vi "Simple Serial.vi"() -> ()   [LabVIEW 2018]
doc: "This example performs a serial port write and a serial port read. The parameters set for the serial port must match the parameters of the connected instrument or device. The VISA Configure Serial Port VI sets the configuration parameters. The front panel displays the controls used to configure the basic parameters, such as baud rate, data bits, and parity. The VI passes the VISA resource name to other VIs that perform operations on that VISA resource. The VISA Write function sends a command to the serial device and the VISA Read function returns data based on the command. The VISA Close function then closes the reference to the serial device. It is important to close the reference; otherwise, further communication through that port might not be possible."
uses:
  <vilib>/Instr/_visa.llb/VISA Configure Serial Port (Instr).vi
panel:
  out "Byte Array stored Every Loop":u8[][](array[numeric])
  out "Current Byte Array":u8[](array[numeric])
  out "ASCII RETURN":string
  in  "Max Read Buffer":i32=100
  in  "stop":bool
  in  "Command":string="MODE?\r"
  in  "Serial Settings":T1={"baud rate"=115200, "data bits"=8, "parity"=enum."None", "stop bits"=10, "flow control"=2} {"flow control" items=["None"=0, "XON/XOFF"=1, "RTS/CTS"=2, "DTR/DSR"=4]; "stop bits" items=["1.0"=10, "1.5"=15, "2.0"=20]; "data bits" min=5 max=8 step=1; "baud rate" items=["75"=75, "110"=110, "134"=134, "150"=150, "300"=300, "600"=600, "1200"=1200, "1800"=1800, "2400"=2400, "4800"=4800, "7200"=7200, "4"=9600, "14400"=14400, "19200"=19200, "28800"=28800, "38400"=38400, "56000"=56000, "57600"=57600, "115200"=115200, "128000"=128000, "230400"=230400]}
  in  "delay before read (ms)":u32=500
  in  "VISA resource name":refnum<visa-resource-name>="COM1"
  # "Overview: Demonstrates the use of NI-VISA for reading USB Time Stamp Counter.  The commands for device is in Wiki. Note that the COUNTS? command must not be in the same command line with other read commands, due to an issue with the termination character."
  # "Note: For an example of how to perform continuous serial communication in a loop, open the Continuous Serial Write and Read.vi in the same folder as this example."
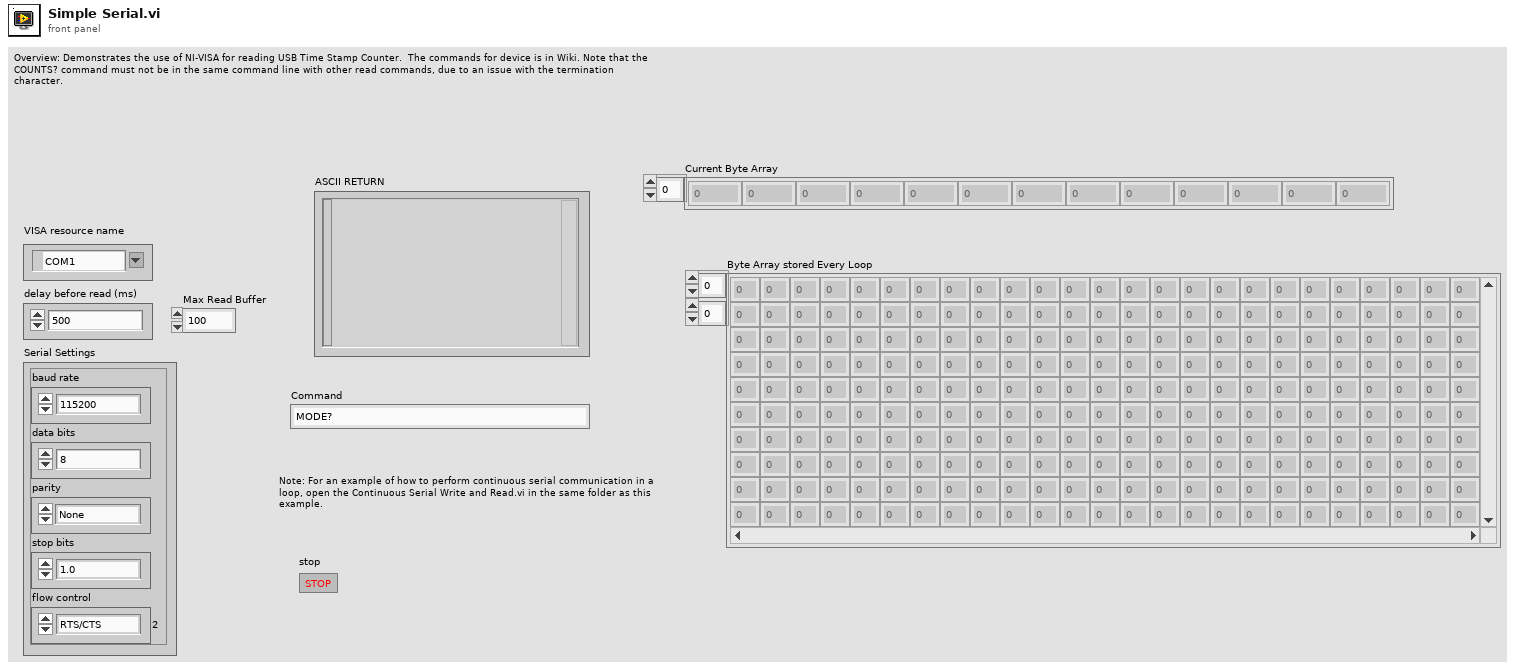
[diagram p1: front panel]
types:
  T1 = cluster{"baud rate":u32, "data bits":u16, "parity":enum16{"None", "Odd", "Even", "Mark", "Space"}, "stop bits":u16, "flow control":u16}
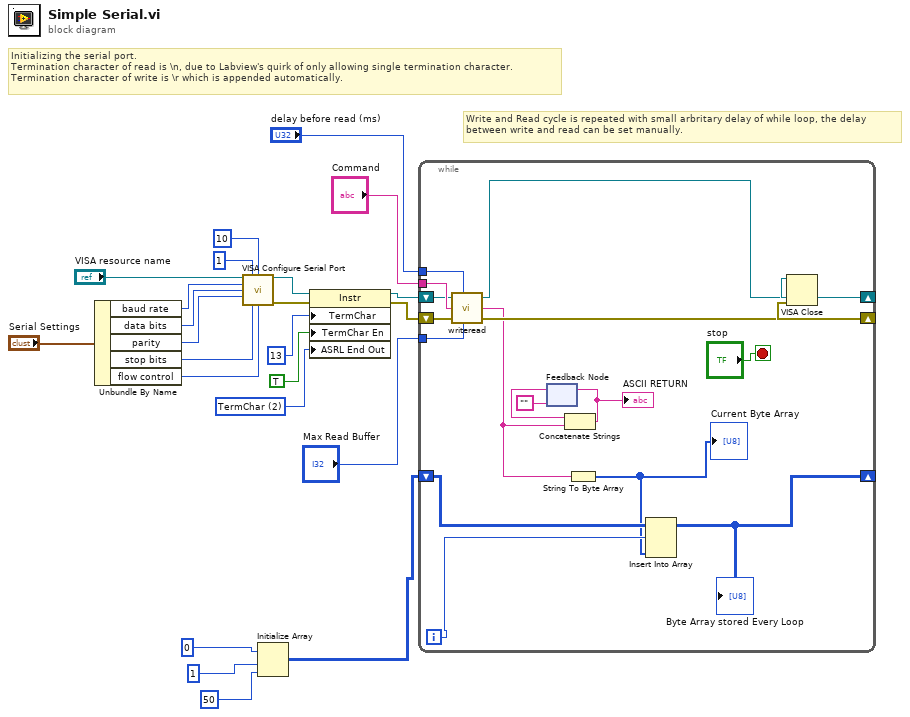
[diagram p0: block diagram]
diagram:
  w5 = u16 2 items=["None", "Last Bit", "TermChar", "Break"] ("Serial Settings:End Mode for Writes")
  # "Write and Read cycle is repeated with small arbritary delay of while loop, the delay \nbetween write and read can be set manually."
  # "Initializing the serial port.\nTermination character of read is \\n, due to Labview's quirk of only allowing single termination character.\nTermination character of write is \\r which is appended automatically."
  n1 = Unbundle By Name("Serial Settings") -> ("baud rate"=w23:u32, "data bits"=w22:u16, "parity"=w21:enum16{"None", "Odd", "Even", "Mark", "Space"}, "stop bits"=w20:u16, "flow control"=w19:u16)
  n2 = call-poly "VISA Configure Serial Port"("VISA resource name"="VISA resource name", "timeout (10sec)"=1, "termination char\n(0xA = '\\n' = LF)"=10, "baud rate (9600)"=w23, "data bits (8)"=w22, "parity (0:none)"=w21, "stop bits (10: 1 bit)"=w20, "flow control (0:none)"=w19) -> ("VISA resource name out"=w11:refnum<visa-resource-name>, "error out"=w9:errorcluster)  [unwired: 2 in, 4 out]
  n3 = Initialize Array(0, 1, 50) -> (w2:i32[][])
  n4 = property class="Instr"(reference=w11, error in=w9, "TermChar"=13, "TermChar En"=TRUE, "ASRL End Out"=w5) -> (reference out=w10:refnum<visa-resource-name>, error out=w8:errorcluster)
  n5 = while {
    tunnel: "delay before read (ms)" -> [w38]
    tunnel: "Command" -> [w37]
    shift-right: [w39] -> w13
    shift-left: w8 -> [w35]
    shift-right: [w40] -> w14
    shift-left: w10 -> [w36]
    tunnel: "Max Read Buffer" -> [w34]
    shift-right: [w26] -> _
    shift-left: w2 -> [w29]
    i -> [w28]
    stop <- "stop" stop-if-true
    n6 = call "writeread.vi"("VISA resource input"=w36, "Read Delay"=w38, "write buffer"=w37, "error in (no error)"=w35, "Max Read Buffer"=w34) -> ("VISA resource out"=w40:refnum<visa-resource-name>, "Response 2"=w30:string, "error out"=w39:errorcluster)  [unwired: 2 in]
    n7 = feedback #1("") -> (w33:string)
    n8 = Concatenate Strings(w33, w30) -> (w31:string)
    "ASCII RETURN" <- w31
    n9 = feedback-in #1(w31) -> ()
    n10 = String To Byte Array(string=w30) -> (unsigned byte array=w27:u8[])
    "Current Byte Array" <- w27
    n11 = Insert Into Array(array=w29, index (row)=w28, new element=w27) -> (w26:i32[][])  [unwired: 1 in]
    "Byte Array stored Every Loop" <- w26
  }
  n12 = VISA Close(VISA resource name=w14, error in (no error)=w13) -> ()  [unwired: 1 out]
